vi "writeToXML.vi"(8 "error in (no error)":errorcluster, 10 "ClassLabel":string, 11 "WavefrontTargetClearOffset in":refnum<class "WavefrontTargetClearOffset.lvclass">) -> (0 "error out":errorcluster, 2 "XML out":string, 3 "WavefrontTargetClearOffset out":refnum<class "WavefrontTargetClearOffset.lvclass">)   [LabVIEW 2014, in "TCSDataDefinitions.lvlib" / "TCSCommand.lvlib" / "OffsetCommands.lvlib" / "WavefrontTargetClearOffset.lvclass"]
uses:
  WavefrontTargetClearOffset.lvclass
  ClearOffset/ClearOffset.lvclass
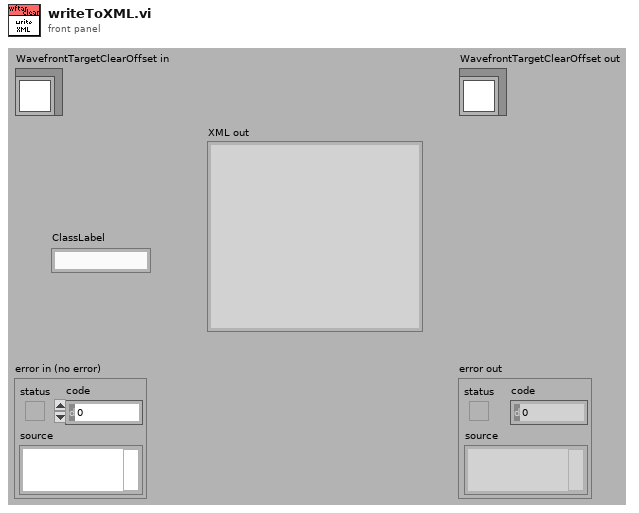
[diagram p1: front panel]
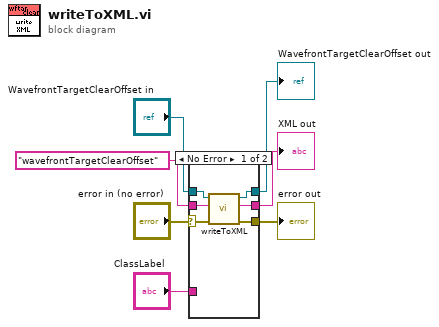
[diagram p0: block diagram]
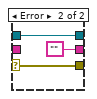
[diagram p2: hidden frame]
diagram:
  n1 = case shown="No Error" "error in (no error)" {
    selector: "error in (no error)" -> [w11 w16]
    tunnel: [w10 w16] -> w6
    tunnel: [w12 w15] -> w4
    tunnel: "WavefrontTargetClearOffset in" -> [w13 w15]
    tunnel: [w9 ""] -> w3
    tunnel: "wavefrontTargetClearOffset" ("ClassLabel") -> [w8 _]
    tunnel: "ClassLabel" -> [_ _]
    frame No Error {
      n2 = call-parent "writeToXML.vi"("error in (no error)"=w11, "ClassLabel"=w8, "ClearOffset in"=w13) -> ("error out"=w10:errorcluster, "XML out"=w9:string, "ClearOffset out"=w12:refnum<class "WavefrontTargetClearOffset.lvclass">)  [unwired: 6 in]
    }
    frame Error {
    }
  }
  "error out" <- w6
  "WavefrontTargetClearOffset out" <- w4
  "XML out" <- w3
